vi "CRYRecall.vi"(0 "Setup in":T1={"No.VI"=0, "Category"="", "StepName"="", "Seq setup flattened"="", "Comment"="", "Steps config."=[], "Jump config"=[], "Start"=0.0, "Increment"=0.0, "Name"="Pa", "Unit"="Pa", "Y data"=1, "Y prefix"="", "Y dB ref"=1.0, "Y unit"="", "Repeat State Array"=[]} {"Repeat State Array"."Start" format="%#_5g"; "Y dB ref" format="%.1f"; "Y data" items=["dB", "Lin"]; "Start" format="%#_5g"}, 5 "Data in":T6 {"Z data" items=["dB", "Lin"]; "X data" items=["dB", "Lin"]; "Y data" items=["dB", "Lin"]; "Z dB ref" format="%.1f"; "Z axis" items=["Log", "Lin"]; "X dB ref" format="%.1f"; "X axis" items=["Log", "Lin"]; "Y axis" items=["Log", "Lin"]; "Y dB ref" format="%.1f"; "Curve"."z" format="%.2f"; "Curve"."y" format="%.2f"; "Curve"."x" format="%.2f"}, 7 "Results in":T2 {"Margin" format="%.2f"}, 9 "Seq Setup in":string, 11 "Step name":string, 12 "Hardware in":string, 13 "Calibration in":string) -> (3 "Types Out":string[](array[string]), 4 "Inserted Names Out":string[](array[string]), 6 "Data out":T6 {"Z data" items=["dB", "Lin"]; "X data" items=["dB", "Lin"]; "Y data" items=["dB", "Lin"]; "Z dB ref" format="%.1f"; "Z axis" items=["Log", "Lin"]; "X dB ref" format="%.1f"; "X axis" items=["Log", "Lin"]; "Y axis" items=["Log", "Lin"]; "Y dB ref" format="%.1f"; "Curve"."z" format="%.2f"; "Curve"."y" format="%.2f"; "Curve"."x" format="%.2f"}, 8 "Results out":T2 {"Margin" format="%.2f"}, 10 "Wave out":T4 {"Y dB ref" format="%.1f"; "Y axis" items=["Log", "Lin"]; "Y data" items=["dB", "Lin"]; "X data" items=["dB", "Lin"]})   [LabVIEW 2013]
uses:
  Typedef Control/CRYData Cluster Array.ctl
  Typedef Control/CRYData Cluster.ctl
  Typedef Control/CRYResult Cluster Array.ctl
  Typedef Control/CRYResult Cluster.ctl
  Typedef Control/CRYWaveform Cluster Array.ctl
  Typedef Control/CRYWaveform Cluster.ctl
  Typedef Control/CRYStep.ctl
  CRYMainGlobal.vi
  SubVI/CRYRecall Global.vi
  Calibration/SubVI/CRYCal Global.vi
  CRYProject/CRYProject Editor Global.vi
  Data/CRYData & result stacks global.vi
  Task Sequence/CRYProject Run Control Global.vi
panel:
  in  "Display Step":bool=TRUE
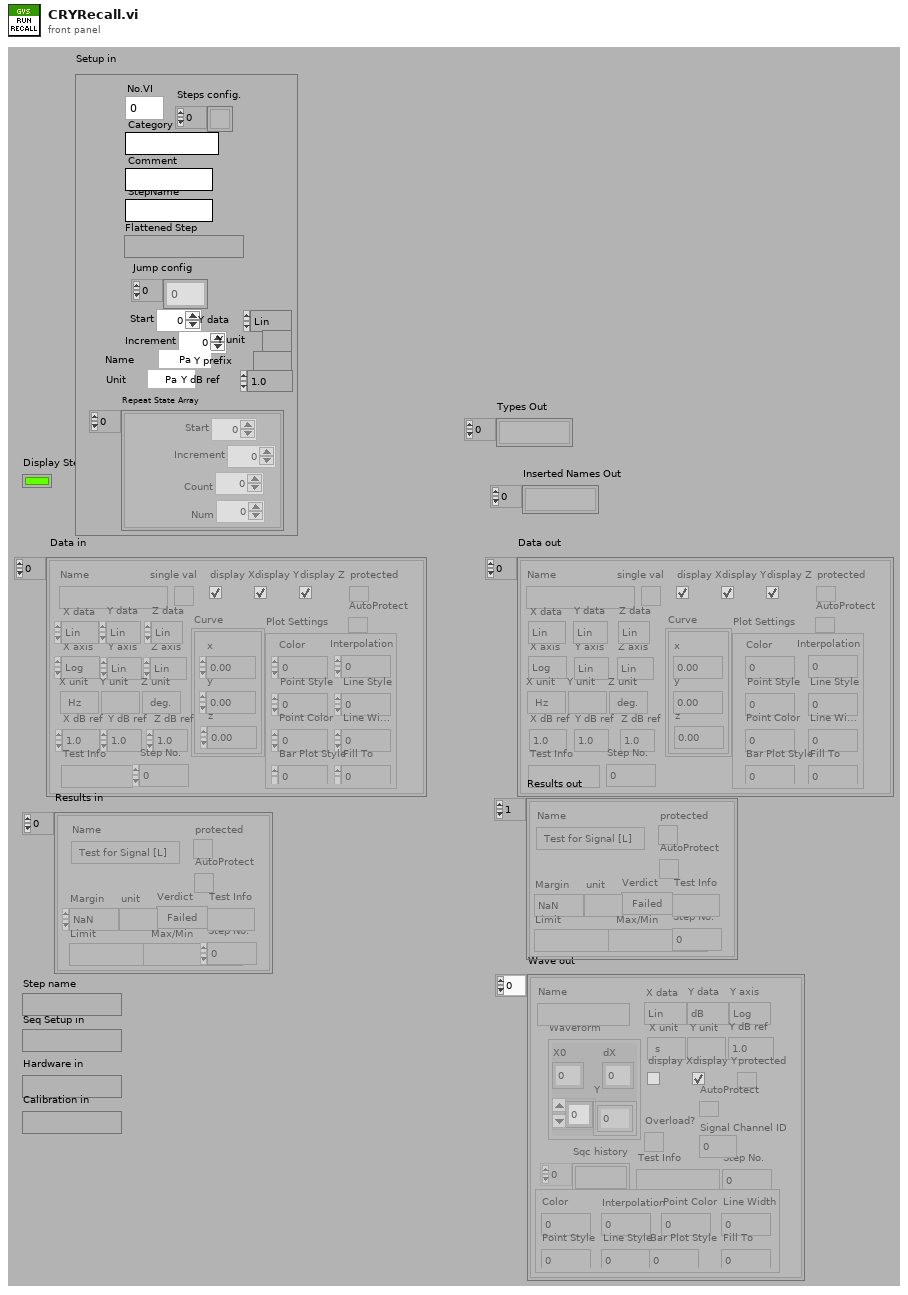
[diagram p1: front panel]
types:
  T1 = typedef "CRYStep.ctl" = cluster{"No.VI":i32, "Category":string, "StepName":string, "Seq setup flattened":string, "Comment":string, "Steps config.":bool[], "Jump config":i32[], "Start":dbl, "Increment":dbl, "Name":string, "Unit":string, "Y data":u16, "Y prefix":string, "Y dB ref":dbl, "Y unit":string, "Repeat State Array":cluster{"Start":dbl, "Increment":dbl, "Count":i32, "Num":i32}[]}
  T2 = typedef "CRYResult Cluster Array.ctl" = T3[]
  T3 = typedef "CRYResult Cluster.ctl" = cluster{"Name":string, "Margin":dbl, "unit":string, "Verdict":bool, "Limit":string, "Max/Min":string, "protected":bool, "Step No.":i32, "Test Info":string, "AutoProtect":bool}
  T4 = typedef "CRYWaveform Cluster Array.ctl" = T5[]
  T5 = typedef "CRYWaveform Cluster.ctl" = cluster{"Waveform":cluster{"X0":dbl, "dX":dbl, "Y":sgl[]}, "X data":u16, "Y data":u16, "Y axis":u16, "X unit":string, "Y unit":string, "Y dB ref":dbl, "display Y":bool, "display X":bool, "Overload?":bool, "Test Info":string, "Step No.":i32, "Name":string, "protected":bool, "Sqc history":string[], "Signal Channel ID":i32, "Plot Settings":cluster{"Color":u32, "Interpolation":u8, "Point Style":u8, "Line Style":u8, "Point Color":u32, "Line Width":u8, "Bar Plot Style":u8, "Fill To":i16}, "AutoProtect":bool}
  T6 = typedef "CRYData Cluster Array.ctl" = T7[]
  T7 = typedef "CRYData Cluster.ctl" = cluster{"Name":string, "Curve":cluster{"x":dbl, "y":dbl, "z":dbl}[], "X data":u16, "Y data":u16, "Z data":u16, "X axis":u16, "Y axis":u16, "Z axis":u16, "X unit":string, "Y unit":string, "Z unit":string, "X dB ref":dbl, "Y dB ref":dbl, "Z dB ref":dbl, "single val":bool, "protected":bool, "display X":bool, "display Y":bool, "display Z":bool, "Test Info":string, "Step No.":i32, "Plot Settings":cluster{"Color":u32, "Interpolation":u8, "Point Style":u8, "Line Style":u8, "Point Color":u32, "Line Width":u8, "Bar Plot Style":u8, "Fill To":i16}, "AutoProtect":bool}
  T8 = cluster{"Start":dbl, "Increment":dbl, "Count":i32, "Num":i32}[]
  T9 = typedef "CRYRecall Cluster.ctl" = cluster{"Name":string, "filepath":string, "all or last":i32, "File Path Mode":u16, "Curve Names":string[], "format string":cluster{"dB Format String out":string, "Lin Format String out":string}, "Template":u16[], "Axis":u16, "*.imp Path":path, "Filepath option":i16, "ML Value":dbl, "user defined":string, "Curves Selected?":bool[], "Help":string, "Tab Value":enum32{"Setting", "Help"}, "Selector":i32, "Use Default":bool}
  T10 = cluster{"dB Format String out":string, "Lin Format String out":string}
  T11 = enum16{"OK", "Yes", "YesNo", "YesNoCancel", "ReplaceAppend"}
  T12 = typedef "CRYTS.ctl" = cluster{"No.TS":u16, "TS File Path":path, "TS Name":string, "EditStepName":string, "Steps":T1[], "New State":bool, "Change State":bool, "Flattened CurveLib Data":string, "Document Data":string, "EditStepNo":u16, "Operator Start File":string, "Sequence Type":string, "Sequence Language":string}
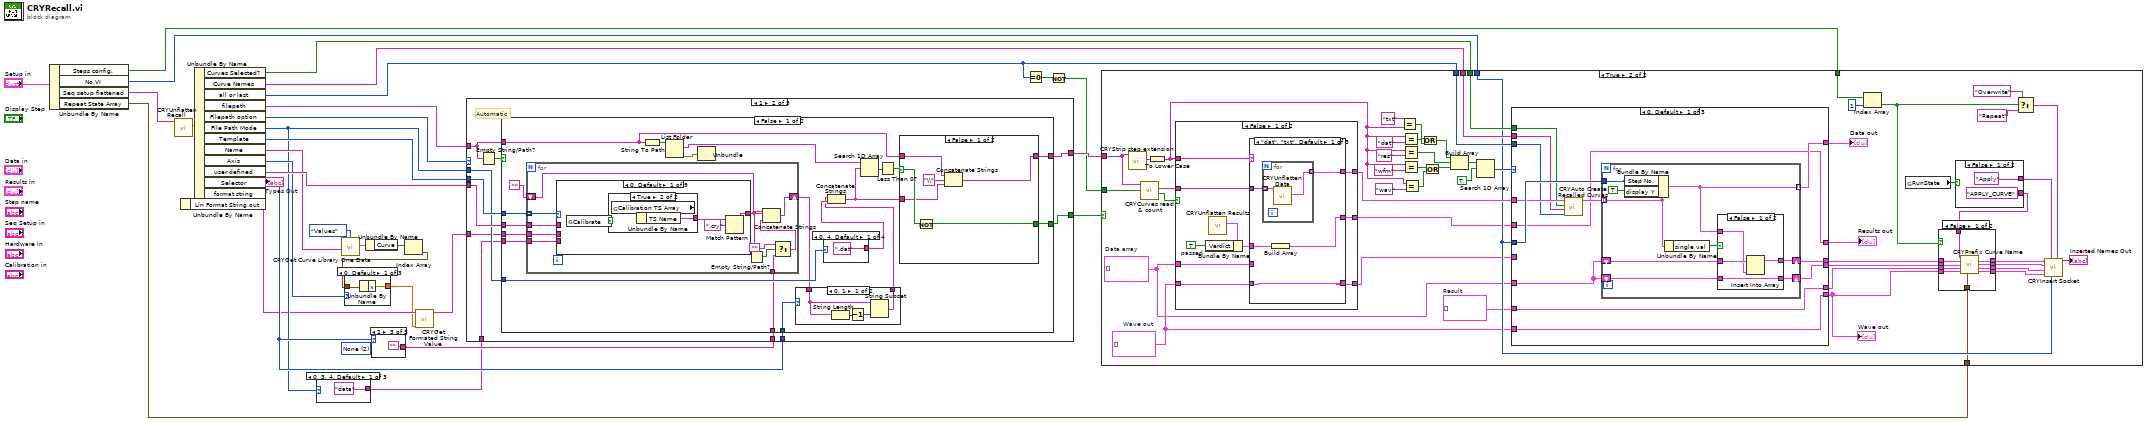
[diagram p0: block diagram]
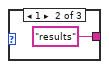
[diagram p2: hidden frame]
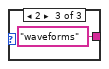
[diagram p3: hidden frame]
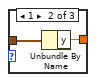
[diagram p4: hidden frame]
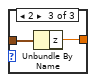
[diagram p5: hidden frame]
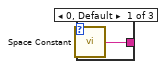
[diagram p6: hidden frame]
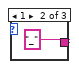
[diagram p7: hidden frame]
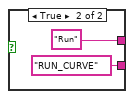
[diagram p9: hidden frame]
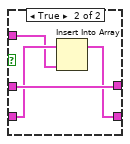
[diagram p11: hidden frame]
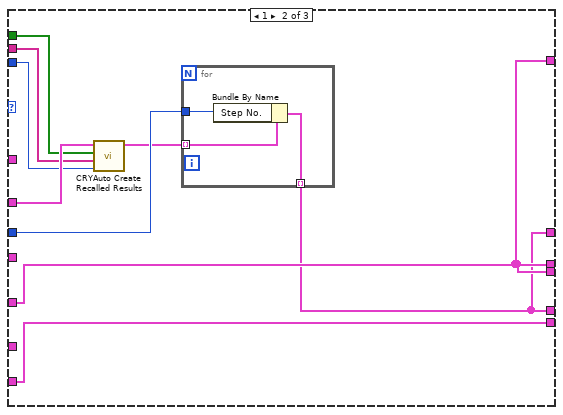
[diagram p12: hidden frame]
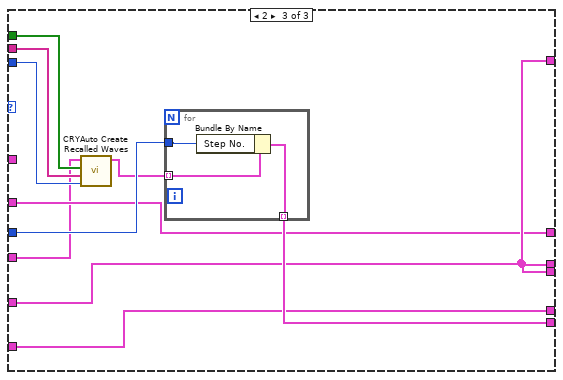
[diagram p13: hidden frame]
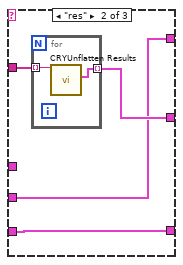
[diagram p14: hidden frame]
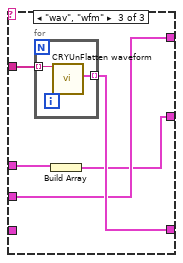
[diagram p15: hidden frame]
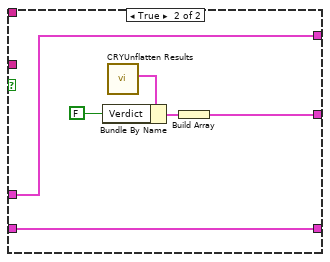
[diagram p16: hidden frame]
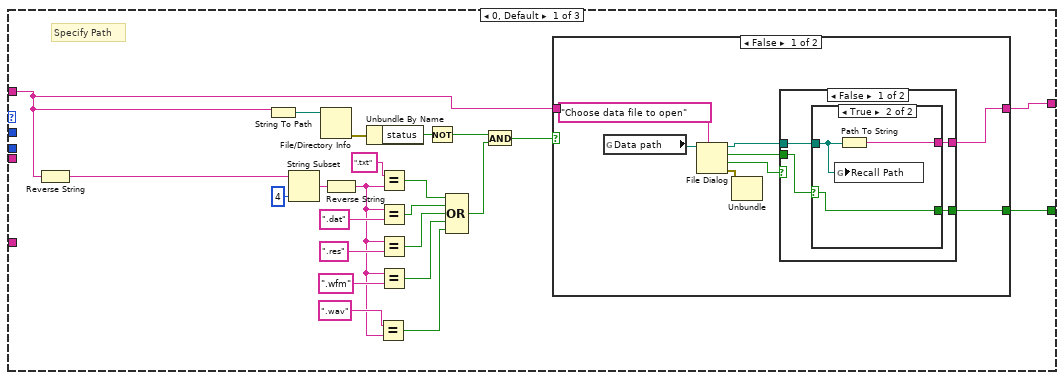
[diagram p17: hidden frame]
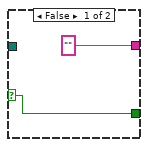
[diagram p18: hidden frame]
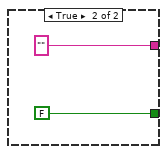
[diagram p19: hidden frame]
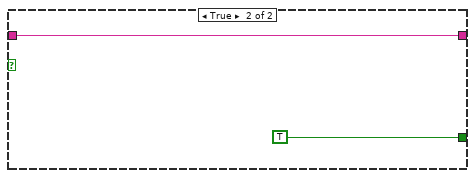
[diagram p20: hidden frame]
diagram:
  (unwired) 2 items=["Space", "Underscores", "None"] ("Selector")
  n1 = Unbundle By Name("Setup in") -> ("Steps config."=w17:bool[], "No.VI"=w18:i32, "Seq setup flattened"=w19:string, "Repeat State Array"=w16:T8)
  n2 = call "CRYUnflatten Recall.vi"("Flatten Recall"=w19) -> ("Recall setup"=w31:T9)  [unwired: 8 in, 2 out]
  n3 = Unbundle By Name(w31) -> ("Curves Selected?"=w24:bool[], "Curve Names"=w25:string[], "all or last"=w23:i32, "filepath"=w30:string, "Filepath option"=w7:i16, "File Path Mode"=w5:u16, "Template"=w27:u16[], "Name"=w9:string, "Axis"=w8:u16, "user defined"=w26:string, "Selector"=w14:i32, "format string"=w4:T10)
  n4 = Unbundle By Name(w4) -> ("Lin Format String out"=w3:string)
  n5 = case shown="0, 3, 4, Default" w5 {
    tunnel: ["data" "results" "waveforms"] -> w6
    frame 0, 3, 4, Default {
    }
    frame 1 {
    }
    frame 2 {
    }
  }
  n6 = call "CRYGet Curve Library One Data .vi"("Data Name"=w9, "Type"=enum16{"Curves", "Values", "Results", "WFM"}."Values") -> ("Value"=w12:T7)  [unwired: 3 in, 6 out]
  n7 = Unbundle By Name(w12) -> ("Curve"=w11:cluster{"x":dbl, "y":dbl, "z":dbl}[])
  n8 = case shown="2" w14 {
    tunnel: [w35 "_" ""] -> w15
    frame 0, Default {
      n9 = call <vilib>:"Space Constant.vi"() -> ("String"=w35:string)
    }
    frame 1 {
    }
    frame 2 {
    }
  }
  n10 = Index Array(array=w11) -> (element=w10:cluster{"x":dbl, "y":dbl, "z":dbl})  [unwired: 1 in]
  n11 = case shown="0, Default" w8 {
    tunnel: w10 -> [w39 w41 w43]
    tunnel: [w38 w40 w42] -> w1
    frame 0, Default {
      n12 = Unbundle By Name(w39) -> ("x"=w38:dbl)
    }
    frame 1 {
      n13 = Unbundle By Name(w41) -> ("y"=w40:dbl)
    }
    frame 2 {
      n14 = Unbundle By Name(w43) -> ("z"=w42:dbl)
    }
  }
  n15 = call "CRYGet Formated String Value.vi"("Value"=w1, "Flattened Format String"=w3) -> ("Unflattened Format string"=w2:string)  [unwired: 9 in]
  n16 = case shown="1" w7 {
    tunnel: w30 -> [w59 w93 _]
    tunnel: [w58 w92 w181] -> w29
    tunnel: [w57 w94 w180] -> w28
    tunnel: w5 -> [_ w95 w179]
    tunnel: w27 -> [_ w97 _]
    tunnel: w26 -> [_ w96 _]
    tunnel: w15 -> [_ w91 _]
    tunnel: w14 -> [_ w90 _]
    tunnel: w2 -> [_ w89 _]
    tunnel: w6 -> [_ w88 _]
    frame 0, Default {
      # "Specify Path"
      n17 = Reverse String(1:w59) -> (0:w66:string)
      n18 = String To Path(string=w59) -> (path=w61:path)
      n19 = String Subset(string=w66, length (rest)=4 ("length (rest)")) -> (substring=w64:string)  [unwired: 1 in]
      n20 = File/Directory Info(path=w61) -> (error out=w62:errorcluster)  [unwired: 1 in, 6 out]
      n21 = Reverse String(1:w64) -> (0:w45:string)
      n22 = Unbundle By Name(w62) -> ("status"=w48:bool)
      n23 = Equal?(x=".wav", y=w45) -> (x = y?=w44:bool)
      n24 = Equal?(x=".txt", y=w45) -> (x = y?=w53:bool)
      n25 = Equal?(x=w45, y=".dat") -> (x = y?=w52:bool)
      n26 = Equal?(x=w45, y=".res") -> (x = y?=w51:bool)
      n27 = Equal?(x=w45, y=".wfm") -> (x = y?=w50:bool)
      n28 = Not(x=w48) -> (.not. x?=w47:bool)
      n29 = Compound Arithmetic op=OR(w53, w52, w51, w50, w44) -> (w49:bool)
      n30 = And(x=w47, y=w49) -> (x .and. y?=w60:bool)
      n31 = case shown="False" w60 {
        tunnel: w59 -> [_ w87]
        tunnel: [w68 w87] -> w58
        tunnel: [w69 TRUE] -> w57
        frame False {
          n32 = global read "CRYMainGlobal.vi" "Data path"() -> (w70:path)
          n33 = File Dialog(7:"Choose data file to open" ("prompt"), 11:w70) -> (0:w72:errorcluster, 1:w73:bool, 2:w74:bool, 3:w67:path)  [unwired: 3 in, 2 out]
          n34 = Unbundle(w72) -> ()  [unwired: 3 out]
          n35 = case shown="False" w73 {
            tunnel: w74 -> [w78 _]
            tunnel: [w77 FALSE] -> w69
            tunnel: w67 -> [w76 _]
            tunnel: [w75 ""] -> w68
            frame False {
              n36 = case shown="True" w78 {
                selector: w78 -> [w80 w83]
                tunnel: [w80 w83] -> w77
                tunnel: w76 -> [_ w81]
                tunnel: ["" w82] -> w75
                frame False {
                }
                frame True {
                  n37 = global write "CRYRecall Global.vi" "Recall Path"(w81) -> ()
                  n38 = Path To String(path=w81) -> (string=w82:string)
                }
              }
            }
            frame True {
            }
          }
        }
        frame True {
        }
      }
    }
    frame 1 {
      # "Automatic"
      n39 = Empty String/Path?(string/path=w93) -> (empty?=w98:bool)
      n40 = case shown="False" w98 {
        tunnel: w95 -> [w118 _]
        tunnel: [w116 FALSE] -> w94
        tunnel: w97 -> [w106 _]
        tunnel: w96 -> [w105 _]
        tunnel: w93 -> [w111 _]
        tunnel: [w112 "" ("filepath")] -> w92
        tunnel: w91 -> [w104 _]
        tunnel: w90 -> [w101 _]
        tunnel: w89 -> [w100 _]
        tunnel: w88 -> [w99 _]
        frame False {
          n41 = for {
            tunnel: w106 -> [w134] mode=indexing
            tunnel: w105 -> [w133]
            shift-right: [w132] -> w103
            shift-left: "" -> [w131]
            tunnel: w104 -> [w128]
            tunnel: w100 -> [w125]
            tunnel: w99 -> [w124]
            n42 = case shown="0, Default" w134 {
              tunnel: [w135 w142 w143 w144 w148 w149 w150 w151 w152] -> w127
              tunnel: w133 -> [_ _ w143 _ _ _ _ _ _]
              tunnel: w125 -> [_ _ _ _ _ _ _ w151 _]
              tunnel: w124 -> [_ _ _ _ _ _ w150 _ _]
              frame 0, Default {
                n43 = global read "CRYCal Global.vi" "Calibrate"() -> (w136:bool)
                n44 = case shown="True" w136 {
                  tunnel: [w139 w140] -> w137
                  frame False {
                    n45 = call "CRYGet Current TS Steps.vi"() -> ("TS Name"=w139:string)  [unwired: 7 in, 4 out]
                  }
                  frame True {
                    n46 = global read "CRYProject Editor Global.vi" "Calibration TS Array"() -> (w141:T12)
                    n47 = Unbundle By Name(w141) -> ("TS Name"=w140:string)
                  }
                }
                n48 = Match Pattern(string=w137, regular expression=".cry") -> (before substring=w135:string)  [unwired: 1 in, 3 out]
              }
              frame 1 {
                n49 = global read "CRYData & result stacks global.vi" "Lot #"() -> (w142:string)
              }
              frame 2 {
              }
              frame 3 {
                n50 = global read "CRYData & result stacks global.vi" "prev Serial #"() -> (w147:string)
                n51 = global read "CRYData & result stacks global.vi" "Serial #"() -> (w146:string)
                n52 = global read "CRYData & result stacks global.vi" "Redo"() -> (w145:bool)
                n53 = Select(t=w147, s=w145, f=w146) -> (s? t:f=w144:string)
              }
              frame 4 {
                n54 = call "CRYGet Date Time.vi"() -> ("date"=w148:string)  [unwired: 10 in, 1 out]
              }
              frame 5 {
                n55 = call "CRYGet Date Time.vi"() -> ("time"=w149:string)  [unwired: 10 in, 1 out]
              }
              frame 6 {
                # "<d or r>"
              }
              frame 7 {
                # "<clval>"
              }
              frame 8 {
                # "<oper>"
                n56 = global read "CRYMainGlobal.vi" "user name"() -> (w152:string)
              }
            }
            n57 = Empty String/Path?(string/path=w127) -> (empty?=w129:bool)
            n58 = Select(t="", s=w129, f=w128) -> (s? t:f=w126:string)
            n59 = Concatenate Strings(w131, w127, w126) -> (w132:string)
          }
          n60 = String To Path(string=w111) -> (path=w114:path)
          n61 = List Folder(path=w114) -> (filenames=w113:string[], error out=w110:errorcluster)  [unwired: 1 in, 4 out]
          n62 = Unbundle(w110) -> ()  [unwired: 3 out]
          n63 = case shown="0, 1" w101 {
            tunnel: w103 -> [w120 w123]
            tunnel: [w119 w123] -> w102
            frame 0, 1 {
              n64 = String Length(string=w120) -> (length=w122:i32)
              n65 = Decrement(x=w122) -> (x-1=w121:i32)
              n66 = String Subset(string=w120, length (rest)=w121) -> (substring=w119:string)  [unwired: 1 in]
            }
            frame Default {
            }
          }
          n67 = case shown="0, 4, Default" w118 {
            tunnel: [".dat" ".res" ".wfm" ".txt"] -> w117
            frame 0, 4, Default {
            }
            frame 1 {
            }
            frame 2 {
            }
            frame 3 {
            }
          }
          n68 = Concatenate Strings(w102, w117) -> (w115:string)
          n69 = Search 1D Array(1D array=w113, element=w115) -> (index of element=w108:i32)  [unwired: 1 in]
          n70 = Less Than 0?(x=w108) -> (x < 0?=w109:bool)
          n71 = case shown="False" w109 {
            selector: w109 -> [w158 _]
            tunnel: [w157 FALSE] -> w116
            tunnel: w115 -> [w154 w171]
            tunnel: [w153 ""] -> w112
            tunnel: w111 -> [w156 _]
            frame False {
              n72 = Not(x=w158) -> (.not. x?=w157:bool)
              n73 = Concatenate Strings(w156, "\\" ("string"), w154) -> (w153:string)
            }
            frame True {
              n74 = call "CRYGet Error Message.vi"("Error No"=5, "Kind"="Recall") -> ("Message"=w161:string)  [unwired: 4 in, 5 out]
              n75 = call "CRYGet Error Message.vi"("Error No"=4, "Kind"="Recall") -> ("Message"=w162:string, "Window Title"=w163:string)  [unwired: 4 in, 4 out]
              n76 = call <vilib>:"Space Constant.vi"() -> ("String"=w160:string)
              n77 = Concatenate Strings(w162, w160, w171, "." ("string"), w160, w161) -> (w165:string)
              n78 = call "CRYMessage Dialog.vi"("Window Title"=w163, "YesNoCancel"=T11."OK", "Message Content"=w165) -> ()  [unwired: 7 in, 2 out]
            }
          }
        }
        frame True {
        }
      }
    }
    frame 2 {
      # "Prompt operator"
      n79 = global read "CRYMainGlobal.vi" "Data path"() -> (w183:path)
      n80 = File Dialog(7:"Select file to recall" ("prompt"), 11:w183) -> (0:w185:errorcluster, 1:w186:bool, 2:w187:bool, 3:w182:path)  [unwired: 3 in, 2 out]
      n81 = Unbundle(w185) -> ()  [unwired: 3 out]
      n82 = case shown="False" w186 {
        tunnel: w187 -> [w192 _]
        tunnel: [w191 FALSE] -> w180
        tunnel: w182 -> [w190 _]
        tunnel: [w189 ""] -> w181
        tunnel: w179 -> [w188 _]
        frame False {
          n83 = case shown="True" w192 {
            selector: w192 -> [w194 _]
            tunnel: [w194 w195] -> w191
            tunnel: w190 -> [_ w201]
            tunnel: ["" w199] -> w189
            tunnel: w188 -> [_ w197]
            frame False {
            }
            frame True {
              n84 = Path To String(path=w201) -> (string=w199:string)
              n85 = global write "CRYRecall Global.vi" "Recall Path"(w201) -> ()
              n86 = call "CRYStrip step extension.vi"("Step name w/ extension"=w199) -> ("Extension (3-letter category)"=w200:string)  [unwired: 7 in, 3 out]
              n87 = To Lower Case(string=w200) -> (all lower case string=w198:string)
              n88 = case shown="\"dat\", Default" w198 {
                tunnel: w197 -> [w213 w216 w223 _ w227]
                tunnel: [w209 w215 w221 FALSE w225] -> w196
                frame "dat", Default {
                  n89 = Equal?(x=w213, y=u16 0) -> (x = y?=w211:bool)
                  n90 = Equal?(x=w213, y=u16 3) -> (x = y?=w210:bool)
                  n91 = Or(x=w211, y=w210) -> (x .or. y?=w209:bool)
                }
                frame "res" {
                  n92 = Equal?(x=w216, y=u16 1) -> (x = y?=w218:bool)
                  n93 = Equal?(x=w216, y=u16 3) -> (x = y?=w217:bool)
                  n94 = Or(x=w218, y=w217) -> (x .or. y?=w215:bool)
                }
                frame "wfm" {
                  n95 = Equal?(x=u16 2, y=w223) -> (x = y?=w221:bool)
                }
                frame "wav" {
                }
                frame "txt" {
                  n96 = Equal?(x=u16 3, y=w227) -> (x = y?=w225:bool)
                }
              }
              n97 = case shown="False" w196 {
                selector: w196 -> [_ w208]
                tunnel: [FALSE w208] -> w195
                frame False {
                  n98 = call "CRYGet Error Message.vi"("Error No"=12, "Kind"="Curves Library") -> ("Message"=w206:string, "Window Title"=w207:string)  [unwired: 4 in, 4 out]
                  n99 = call "CRYMessage Dialog.vi"("Window Title"=w207, "YesNoCancel"=T11."OK", "Message Content"=w206) -> ()  [unwired: 7 in, 2 out]
                }
                frame True {
                }
              }
            }
          }
        }
        frame True {
        }
      }
    }
  }
  n100 = Equal To 0?(x=w23) -> (x = 0?=w22:bool)
  n101 = Not(x=w22) -> (.not. x?=w21:bool)
  n102 = case shown="True" w28 {
    tunnel: w29 -> [_ w246]
    tunnel: w25 -> [_ w278]
    tunnel: w23 -> [_ w277]
    tunnel: w24 -> [_ w276]
    tunnel: w21 -> [_ w275]
    tunnel: w18 -> [_ w262]
    tunnel: w17 -> [_ w258]
    tunnel: w16 -> [_ w234]
    frame False {
    }
    frame True {
      w249 = T6 []  # Data array
      w254 = T4 []  # Wave out
      w256 = T3[] []  # Result
      n103 = call "CRYStrip step extension.vi"("Step name w/ extension"=w246) -> ("Extension (3-letter category)"=w247:string)  [unwired: 7 in, 3 out]
      n104 = call "CRYCurves read & count.vi"("Last curve only (F)"=w275, "Data file path"=w246) -> ("Canceled"=w280:bool, "Data curves array"=w281:string[])  [unwired: 6 in, 2 out]
      n105 = To Lower Case(string=w247) -> (all lower case string=w245:string)
      n106 = case shown="False" w280 {
        tunnel: w281 -> [w364 _]
        tunnel: [w363 w390] -> w271
        tunnel: [w362 w387] -> w251
        tunnel: w249 -> [w361 w390]
        tunnel: w254 -> [w360 w385]
        tunnel: [w359 w385] -> w248
        tunnel: w245 -> [w355 _]
        frame False {
          w358 = TRUE  # passed
          n107 = call "CRYUnflatten Results.vi"() -> ("Result"=w357:T3)  [unwired: 9 in, 2 out]
          n108 = Bundle By Name(cluster=w357, "Verdict"=w358) -> (w356:T3)
          n109 = case shown="\"dat\", \"txt\", Default" w355 {
            tunnel: w364 -> [w369 w375 w382]
            tunnel: [w368 w373 w380] -> w363
            tunnel: [w367 w374 w378] -> w362
            tunnel: w361 -> [_ w373 w380]
            tunnel: w360 -> [w366 w372 _]
            tunnel: [w366 w372 w381] -> w359
            tunnel: w356 -> [w365 _ w379]
            frame "dat", "txt", Default {
              n110 = for {
                tunnel: w369 -> [w371] mode=indexing
                tunnel: [w370] -> w368 mode=indexing
                n111 = call "CRYUnflatten Data.vi"("Unflatten data"=w371) -> ("Datum"=w370:T7)  [unwired: 8 in, 2 out]
              }
              n112 = Build Array(w365) -> (w367:T3[])
            }
            frame "res" {
              n113 = for {
                tunnel: w375 -> [w377] mode=indexing
                tunnel: [w376] -> w374 mode=indexing
                n114 = call "CRYUnflatten Results.vi"("Unflatten Result"=w377) -> ("Result"=w376:T3)  [unwired: 8 in, 2 out]
              }
            }
            frame "wav", "wfm" {
              n115 = for {
                tunnel: w382 -> [w384] mode=indexing
                tunnel: [w383] -> w381 mode=indexing
                n116 = call "CRYUnFlatten waveform.vi"("Unflatten Waveform"=w384) -> ("Waveform Cluster"=w383:T5)  [unwired: 8 in, 2 out]
              }
              n117 = Build Array(w379) -> (w378:T3[])
            }
          }
        }
        frame True {
          n118 = call "CRYUnflatten Results.vi"() -> ("Result"=w388:T3)  [unwired: 9 in, 2 out]
          n119 = Bundle By Name(cluster=w388, "Verdict"=FALSE) -> (w386:T3)
          n120 = Build Array(w386) -> (w387:T3[])
        }
      }
      n121 = Equal?(x="txt", y=w245) -> (x = y?=w265:bool)
      n122 = Equal?(x=w245, y="dat") -> (x = y?=w264:bool)
      n123 = Equal?(x=w245, y="res") -> (x = y?=w268:bool)
      n124 = Equal?(x=w245, y="wfm") -> (x = y?=w267:bool)
      n125 = Equal?(x=w245, y="wav") -> (x = y?=w252:bool)
      n126 = Or(x=w265, y=w264) -> (x .or. y?=w263:bool)
      n127 = Or(x=w267, y=w252) -> (x .or. y?=w253:bool)
      n128 = Build Array(w263, w268, w253) -> (w269:bool[])
      n129 = Search 1D Array(1D array=w269, element=TRUE) -> (index of element=w266:i32)  [unwired: 1 in]
      n130 = case shown="0, Default" w266 {
        tunnel: w271 -> [w311 _ _]
        tunnel: w278 -> [w308 w334 w348]
        tunnel: w262 -> [w312 w338 w351]
        tunnel: w251 -> [w300 w337 w343]
        tunnel: w277 -> [w307 w333 w347]
        tunnel: w276 -> [w309 w335 w349]
        tunnel: [w306 w332 w345] -> w243
        tunnel: [w305 w332 w345] -> w242
        tunnel: [w301 w330 w344] -> w241
        tunnel: [w302 w331 w346] -> w240
        tunnel: w249 -> [w304 w332 w345]
        tunnel: [w303 w332 w345] -> w257
        tunnel: w256 -> [w301 _ w344]
        tunnel: w254 -> [w302 w331 _]
        tunnel: [w300 w330 w343] -> w250
        tunnel: w248 -> [_ _ w342]
        frame 0, Default {
          n131 = call "CRYAuto Create Recalled Curves.vi"("all or last"=w307, "Curve Names in"=w308, "Curves Selected?"=w309, "Data Array"=w311) -> ("Data Out"=w310:T7[])  [unwired: 7 in]
          n132 = for {
            tunnel: w310 -> [w320] mode=indexing
            tunnel: w312 -> [w321]
            tunnel: [w313] -> w303 mode=indexing
            shift-right: [w316] -> w306
            shift-left: w304 -> [w317]
            shift-right: [w315] -> w305
            shift-left: w304 -> [w314]
            n133 = Bundle By Name(cluster=w320, "Step No."=w321, "display Y"=TRUE) -> (w313:T7)
            n134 = Unbundle By Name(w320) -> ("single val"=w318:bool)
            n135 = case shown="False" w318 {
              tunnel: w313 -> [w323 w327]
              tunnel: w317 -> [w324 w329]
              tunnel: [w322 w329] -> w316
              tunnel: [w325 w326] -> w315
              tunnel: w314 -> [w325 w328]
              frame False {
                n136 = Insert Into Array(array=w324, new element=w323) -> (w322:T6)  [unwired: 1 in]
              }
              frame True {
                n137 = Insert Into Array(array=w328, new element=w327) -> (w326:T6)  [unwired: 1 in]
              }
            }
          }
        }
        frame 1 {
          n138 = call "CRYAuto Create Recalled Results.vi"("all or last"=w333, "Curve Names in"=w334, "Curves Selected?"=w335, "Result Array"=w337) -> ("Resut Out"=w336:T3[])  [unwired: 7 in]
          n139 = for {
            tunnel: w336 -> [w340] mode=indexing
            tunnel: w338 -> [w341]
            tunnel: [w339] -> w330 mode=indexing
            n140 = Bundle By Name(cluster=w340, "Step No."=w341) -> (w339:T3)
          }
        }
        frame 2 {
          n141 = call "CRYAuto Create Recalled Waves.vi"("all or last"=w347, "Curve Names in"=w348, "Curves Selected?"=w349, "Wave array"=w342) -> ("Wave Out"=w350:T5[])  [unwired: 7 in]
          n142 = for {
            tunnel: w350 -> [w352] mode=indexing
            tunnel: w351 -> [w354]
            tunnel: [w353] -> w346 mode=indexing
            n143 = Bundle By Name(cluster=w352, "Step No."=w354) -> (w353:T5)
          }
        }
      }
      "Data out" <- w257
      "Results out" <- w250
      "Wave out" <- w240
      n144 = Index Array(array=w258, index=1) -> (element=w235:bool)
      n145 = global read "CRYProject Run Control Global.vi" "RunState"() -> (w233:bool)
      n146 = case shown="False" w233 {
        tunnel: ["Apply" ("sOption1") "Run" ("Type In")] -> w232
        tunnel: ["APPLY_CURVE" ("Type In") "RUN_CURVE" ("Type In")] -> w231
        frame False {
        }
        frame True {
        }
      }
      n147 = case shown="False" w235 {
        tunnel: w243 -> [w295 w299]
        tunnel: w242 -> [w294 w298]
        tunnel: w241 -> [w293 w297]
        tunnel: w240 -> [w292 w296]
        tunnel: [w291 w299] -> w239
        tunnel: [w290 w298] -> w238
        tunnel: [w289 w297] -> w237
        tunnel: [w288 w296] -> w236
        tunnel: w234 -> [w287 _]
        tunnel: w231 -> [w286 _]
        frame False {
          n148 = call "CRYPrefix Curve Name.vi"("Type In"=w286, "Curves In"=w295, "Values In"=w294, "Results In"=w293, "Waves In"=w292, "Repeat State Array In"=w287) -> ("Curves Out"=w291:T6, "Values Out"=w290:T6, "Results Out"=w289:T2, "Waves Out"=w288:T4)  [unwired: 6 in]
        }
        frame True {
        }
      }
      n149 = Select(t="Overwrite" ("Y unit"), s=w235, f="Repeat") -> (s? t:f=w259:string)
      n150 = call "CRYInsert Socket.vi"("sOption2"=w259, "Step No."=w262, "sOption1"=w232, "Waves"=w236, "Results"=w237, "Values"=w238, "Curves"=w239) -> ("Inserted Names Out"=→"Inserted Names Out":string[])  [unwired: 4 in]
    }
  }
